vi "Task - Pressure & Flow.vi"() -> ()   [LabVIEW 2013]
uses:
  <vilib>/Utility/error.llb/DialogType.ctl
  Global - Pressure & Flow.vi
  <vilib>/Utility/file.llb/Write To Spreadsheet File (DBL).vi
panel:
  in  "MilliSec per Cycle":i32=250
  in  "#Cycles":i32=100000
  out "Temperature (K)":dbl=2.13410741378
  out "Output Pressure":dbl=33.964
  out "Vapor Pressure":T1(graph)={"Pressure value"=33.964, "Converted Output"=2.13410741378}
  out "Pressure (Torr)":dbl=34.2
  in  "MKS 670 Hi-res P":refnum<visa-resource-name>="COM6"
  in  "error in (no error)":errorcluster
  out "error out":errorcluster={"status"=FALSE, "code"=3003, "source"="Task1 completed OK at 100 cycles"}
  out "Time Stamp":timestamp=timestamp(3561144723.7158904 s since 1904-01-01)
  out "stop":bool=TRUE
  out "Heartbeat":bool
  out "Finished":bool=TRUE
  out "Cycle":i32=101
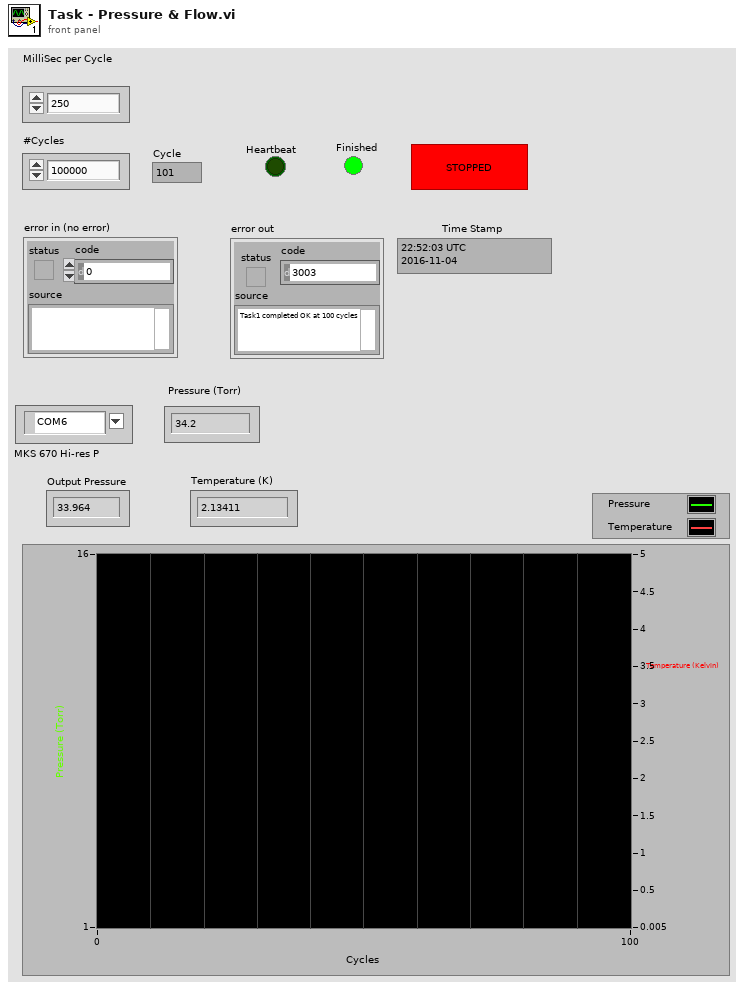
[diagram p1: front panel]
types:
  T1 = cluster{"Pressure value":dbl, "Converted Output":dbl}
  T2 = enum16{"MKS946 High Pressure Gauge", "MKS946 Separator Flow", "MKS946 Target Cavity Flow", "MKS670 Low Pressure Gauge"}
  T3 = typedef "DialogType.ctl" = u16
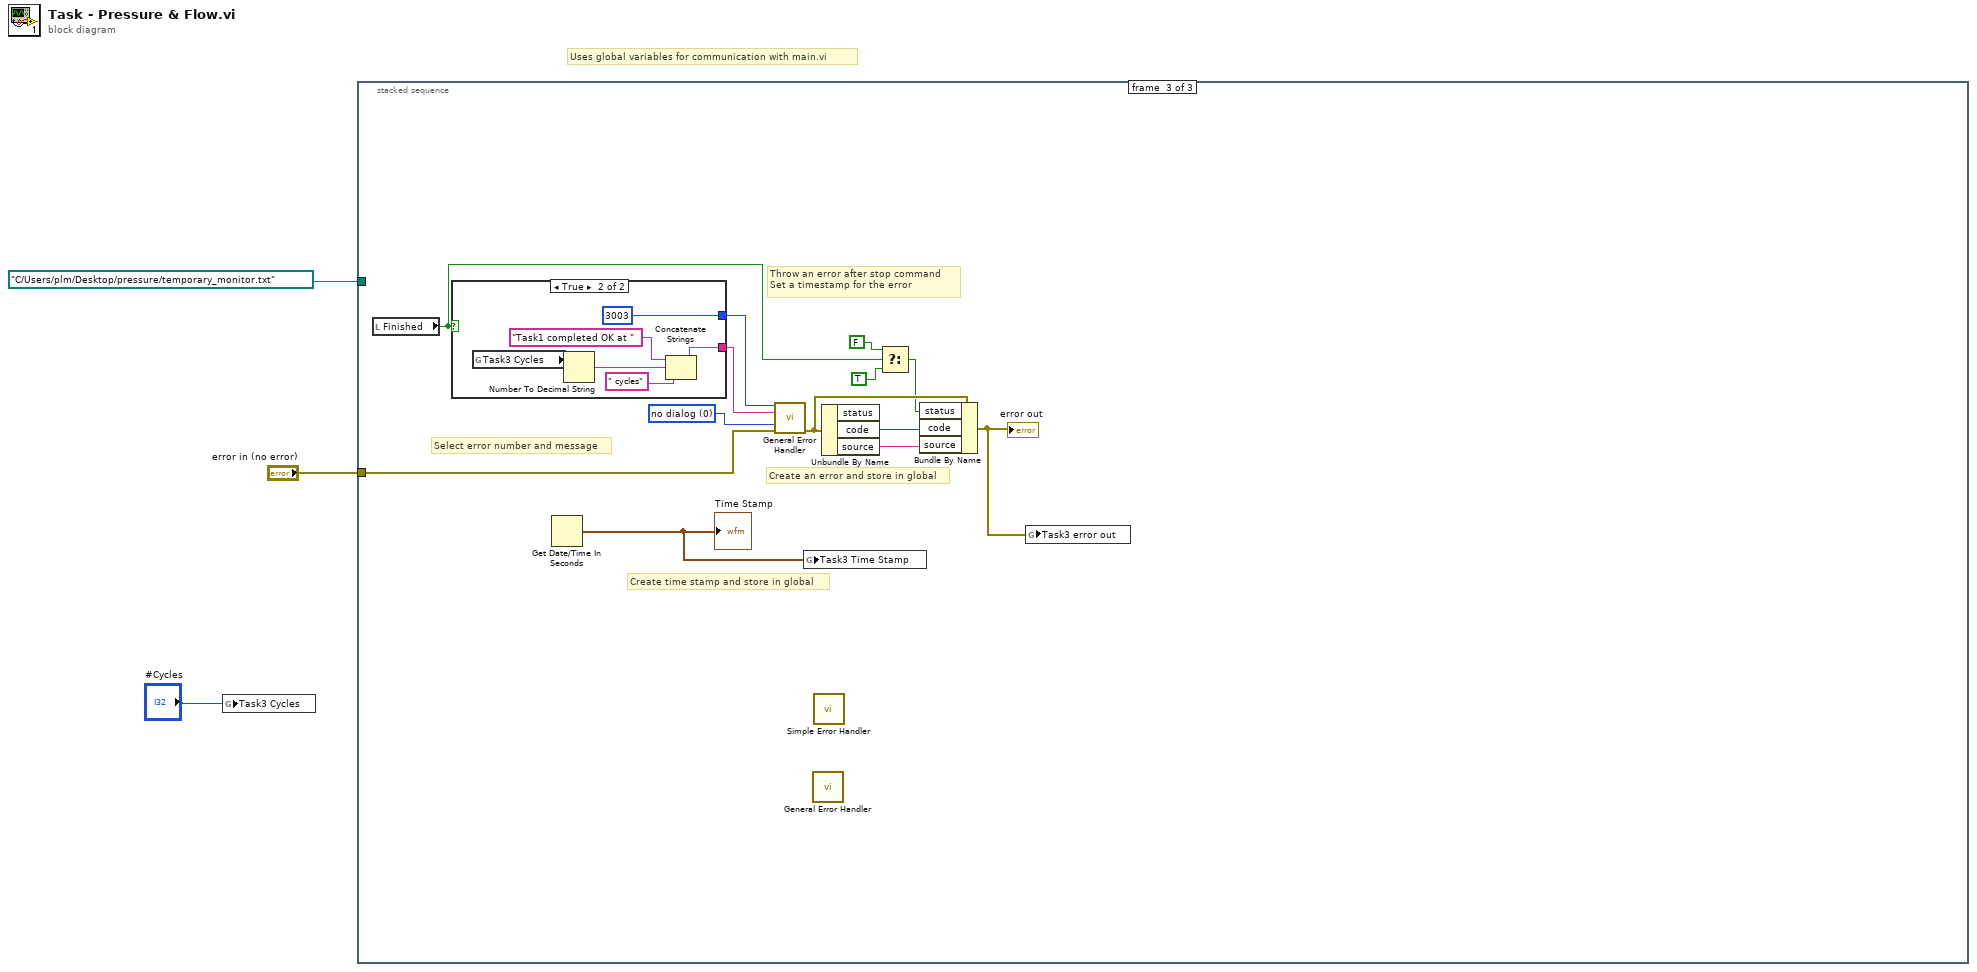
[diagram p0: block diagram]
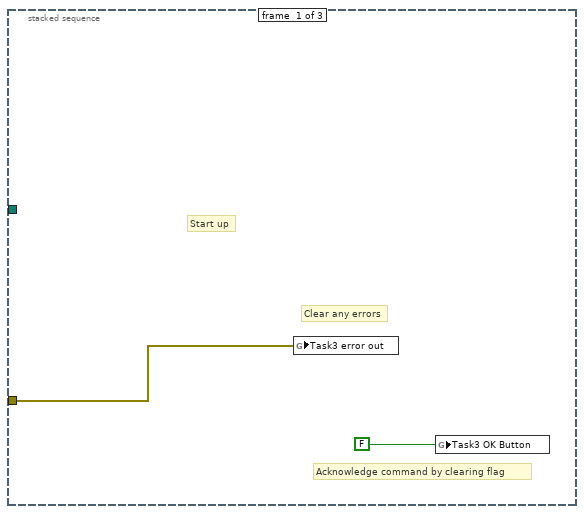
[diagram p2: hidden frame]
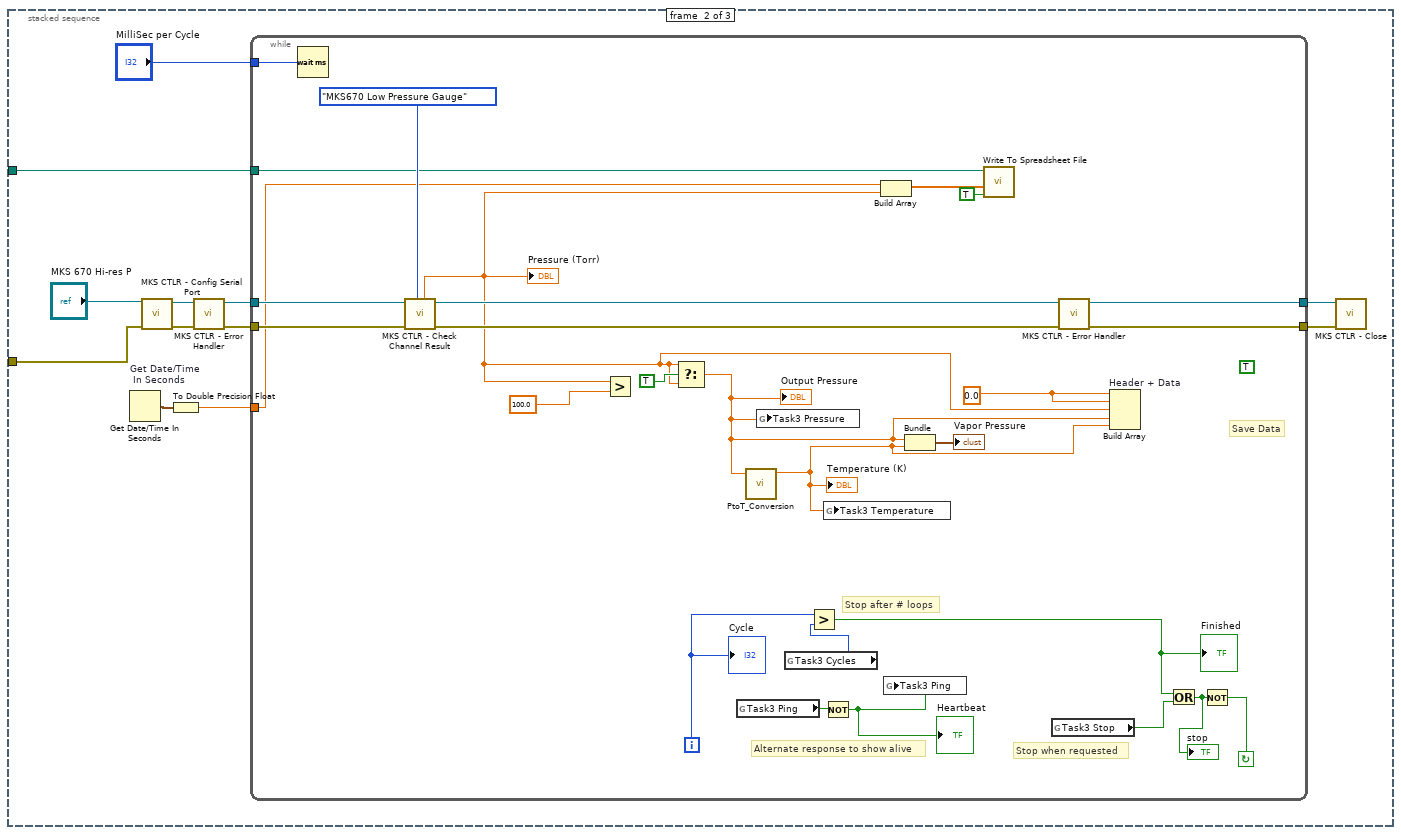
[diagram p3: hidden frame]
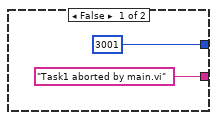
[diagram p4: hidden frame]
diagram:
  # "Uses global variables for communication with main.vi"
  n1 = global write "Global - Pressure & Flow.vi" "Task3 Cycles"("#Cycles") -> ()
  n2 = stacked-sequence {
    tunnel: "error in (no error)" -> [w5 w17 w56]
    tunnel: path "C:/Users/plm/Desktop/pressure/temporary_monitor.txt" ("file path (dialog if empty)") -> [_ w6 _]
    frame #0 {
      # "Start up"
      # "Acknowledge command by clearing flag"
      # "Clear any errors"
      n3 = global write "Global - Pressure & Flow.vi" "Task3 error out"(w5) -> ()
      n4 = global write "Global - Pressure & Flow.vi" "Task3 OK Button"(FALSE) -> ()
    }
    frame #1 {
      n5 = Get Date/Time In Seconds "Get Date/Time\n In Seconds"() -> (seconds since 1Jan1904=w10:timestamp)
      n6 = call "MKS CTLR - Config Serial Port.vi"("Error In"=w17, "MKS ViiSA resource name in"="MKS 670 Hi-res P") -> ("Error Out"=w13:errorcluster, "VISA resource name out"=w12:refnum<visa-resource-name>)  [unwired: 8 in]
      n7 = To Double Precision Float(number=w10) -> (double precision float=w9:dbl)
      n8 = call "MKS CTLR - Error Handler.vi"("error in (no error)"=w13, "VISA resource name (IN)"=w12) -> ("error out"=w14:errorcluster, "VISA resource name (OUT)"=w15:refnum<visa-resource-name>)  [unwired: 8 in]
      n9 = while {
        tunnel: w15 -> [w30]
        tunnel: w14 -> [w31]
        tunnel: [w33] -> w16
        tunnel: [w32] -> w8
        tunnel: "MilliSec per Cycle" -> [w29]
        tunnel: w9 -> [w21]
        tunnel: w6 -> [w22]
        i -> [w37]
        stop <- w44 continue-if-true
        w23 = 0.0
        (unwired) TRUE ("Save Data to File")
        # "Save Data"
        # "Stop after # loops"
        # "Alternate response to show alive"
        # "Stop when requested"
        n10 = Wait (ms)(milliseconds to wait=w29) -> ()  [unwired: 1 out]
        n11 = call "MKS CTLR - Check Channel Result.vi"("Channel"=T2."MKS670 Low Pressure Gauge", "error in (no error)"=w31, "VISA resource name (IN)"=w30) -> ("error out"=w24:errorcluster, "VISA resource name (OUT)"=w25:refnum<visa-resource-name>, "Pressure value"=w20:dbl)  [unwired: 5 in, 1 out]
        "Pressure (Torr)" <- w20
        n12 = Greater?(x=w20, y=100.0) -> ()  [unwired: 1 out]
        n13 = Select(t=w20, s=TRUE, f=w20) -> (s? t:f=w27:dbl)
        "Output Pressure" <- w27
        n14 = global read "Global - Pressure & Flow.vi" "Task3 Ping"() -> (w43:bool)
        n15 = call "PtoT_Conversion.vi"("A"=w27) -> ("Converted Output"=w28:dbl)  [unwired: 9 in, 1 out]
        "Temperature (K)" <- w28
        n16 = global write "Global - Pressure & Flow.vi" "Task3 Pressure"(w27) -> ()
        n17 = global read "Global - Pressure & Flow.vi" "Task3 Cycles"() -> (w38:i32)
        n18 = Greater?(x=w37, y=w38) -> (0:w40:bool)
        "Finished" <- w40
        n19 = Not(x=w43) -> (.not. x?=w42:bool)
        "Heartbeat" <- w42
        n20 = global write "Global - Pressure & Flow.vi" "Task3 Temperature"(w28) -> ()
        n21 = Build Array(w21, w20) -> (w19:dbl[])
        n22 = global write "Global - Pressure & Flow.vi" "Task3 Ping"(w42) -> ()
        n23 = Bundle("Pressure value"=w27, "Converted Output"=w28) -> (→"Vapor Pressure":T1)  [unwired: 1 in]
        n24 = call-poly <vilib>:"Write To Spreadsheet File.vi"("append to file? (new file:F)"=TRUE, "1D data"=w19, "file path (dialog if empty)"=w22) -> ()  [unwired: 5 in, 1 out]
        n25 = global read "Global - Pressure & Flow.vi" "Task3 Stop"() -> (w41:bool)
        n26 = call "MKS CTLR - Error Handler.vi"("error in (no error)"=w24, "VISA resource name (IN)"=w25) -> ("error out"=w32:errorcluster, "VISA resource name (OUT)"=w33:refnum<visa-resource-name>)  [unwired: 8 in]
        n27 = Build Array "Header + Data"(w23, w23, w20, w27, w28) -> ()  [unwired: 1 out]
        n28 = Or(x=w40, y=w41) -> (x .or. y?=w39:bool)
        "stop" <- w39
        n29 = Not(x=w39) -> (.not. x?=w44:bool)
        "Cycle" <- w37
      }
      n30 = call "MKS CTLR - Close.vi"("error in (no error)"=w8, "VISA resource name (IN)"=w16) -> ()  [unwired: 9 in, 1 out]
    }
    frame #2 {
      w57 = T3 0 items=["no dialog", "OK message", "continue or stop message", "OK message + warnings", "continue/stop + warnings"] ("type of dialog (OK msg:1)")
      # "Create time stamp and store in global"
      # "Select error number and message"
      # "Throw an error after stop command\nSet a timestamp for the error"
      # "Create an error and store in global"
      n31 = local read "Finished"() -> (w52:bool)
      n32 = case shown="True" w52 {
        tunnel: [3001 ("[error code] (0)") 3003 ("[error code] (0)")] -> w53
        tunnel: ["Task1 aborted by main.vi" ("[error source] (\" \")") w60] -> w54
        frame False {
        }
        frame True {
          n33 = global read "Global - Pressure & Flow.vi" "Task3 Cycles"() -> (w64:i32)
          n34 = Number To Decimal String(number=w64) -> (decimal integer string=w62:string)  [unwired: 1 in]
          n35 = Concatenate Strings("Task1 completed OK at " ("[error source] (\" \")"), w62, " cycles") -> (w60:string)
        }
      }
      n36 = Get Date/Time In Seconds() -> (seconds since 1Jan1904=w55:timestamp)
      "Time Stamp" <- w55
      n37 = call <vilib>:"General Error Handler.vi"("[error code] (0)"=w53, "[error source] (\" \")"=w54, "type of dialog (OK msg:1)"=w57, "error in (no error)"=w56) -> ("error out"=w47:errorcluster)  [unwired: 7 in, 4 out]
      n38 = global write "Global - Pressure & Flow.vi" "Task3 Time Stamp"(w55) -> ()
      n39 = call <vilib>:"General Error Handler.vi"() -> ()  [unwired: 11 in, 5 out]
      n40 = call <vilib>:"Simple Error Handler.vi"() -> ()  [unwired: 5 in, 5 out]
      n41 = Unbundle By Name(w47) -> ("code"=w49:i32, "source"=w48:string)  [unwired: 1 out]
      n42 = Select(t=FALSE, s=w52, f=TRUE) -> (s? t:f=w45:bool)
      n43 = Bundle By Name(cluster=w47, "status"=w45, "code"=w49, "source"=w48) -> (w46:errorcluster)
      "error out" <- w46
      n44 = global write "Global - Pressure & Flow.vi" "Task3 error out"(w46) -> ()
    }
  }
